vi "FTW-Test-Socket-Stress-InboxConnector.vi"() -> (0 "Test Result":errorcluster)   [LabVIEW 2014]
uses:
  src/socket/support/FTW-Socket-Core-TransportScheme.ctl
  src/error/FTW-ERR-ExceptionType.ctl
  src/error/FTW-ERR-ThrowError.vi
  lib/FTW-KernelFilepath.vi
  src/error/FTW-ERR-CallChain.vi
  src/string/FTW-STR-ReplaceWhitespace.vi
  src/json/core/FTW-JSON-Core-EncodingFlags.vi
  src/reflection/FTW-Reflection-Type.vi
  codegen/xnode/json/fetch/FTW-JSON-Core-GetFlattenedValue.vi
  src/socket/support/FTW-Socket-Core-LibraryError.vi
  src/actor/request/FTW-Request-InterpretResponse.vi
  codegen/xnode/FTW-Actor-Ask.xnode
  src/socket/connector/core/FTW-Connector-Core-Type.ctl
  codegen/xnode/FTW-JSON-Fetch.xnode
panel:
  in  "Mode":enum32{"Automated Testing", "Manual Control"}(tab)
  out "Progress":dbl(slide) scale=0.0..1.0
  in  "Test to Perform":T1(radio)=enum."Parallel: 10x100x10k"
  in  "stop":bool
  out "Results":T3(array[cluster]) {"?" format="%_3p bytes/sec (one-way receive)"; "?" format="%_3f replies/sec"; "?" format="Benchmark Time: %_3psec"}
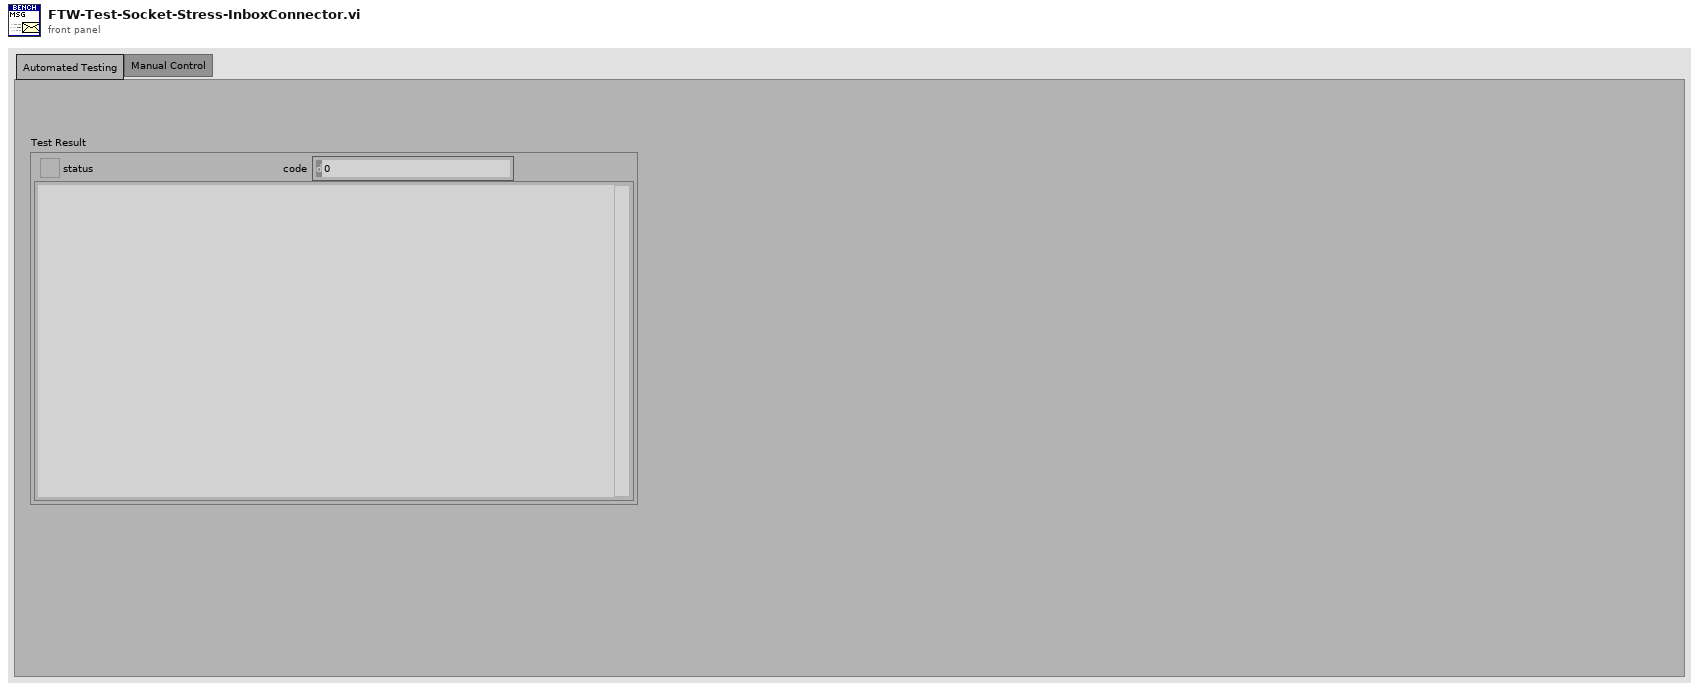
[diagram p1: front panel]
types:
  T1 = enum32{"Serial: 1x1x0", "Serial: 1x1000x0", "Serial: 1x1000x10k", "Serial: 10x100x10k", "Parallel: 10x100x10k", "Parallel: 10x10x1M", "Parallel: 100x1x10k", "Parallel: 100x100x0", "Parallel: 1000x10x1k", "Parallel: 1000x100x10k", "Parallel: 10x100x1M", "Parallel: 1000x1x1M", "Parallel: 10x10000x0"}
  T2 = typedef "FTW-Socket-Core-TransportScheme.ctl" = enum16{"TCP (tcp://)", "Inter-Process (ipc://)", "In-Process (inproc://)", "WebSocket (ws://)"}
  T3 = cluster{"Server Address":T2, "error":errorcluster, "Client Results":cluster{"Instance":string, "All replies were as expected?":bool}[], dbl, dbl, dbl, "Pass?":bool}[]
  T4 = enum32{"Serial: 1x1x0", "Serial: 1x1000x0", "Serial: 1x1000x10k", "Serial: 10x100x10k", "Parallel: 10x100x10k", "Parallel: 10x10x1M", "Parallel: 100x1x10k", "Parallel: 100x100x0", "Parallel: 1000x10x1k", "Parallel: 1000x100x10k", "Parallel: 10x100x1M", "Parallel: 1000x1x1M", "Parallel: 10x10000x0"}[]
  T5 = cluster{"Inbox Address":T2, "error out":errorcluster, cluster{string, bool}[], "Elapsed Time":dbl, dbl, dbl, bool}[]
  T6 = typedef "FTW-ERR-ExceptionType.ctl" = enum16{"OK", "Info", "Warning", "Error"}
  T7 = cluster{i32, i32, i32, i32, "Replies from Server":i32, "bytes from Server":i32, bool, bool}
  T8 = cluster{"Message Transport Scheme":T2, "error out":errorcluster, cluster{string, bool}[], "Elapsed Time":dbl, dbl, dbl, bool}
  T9 = cluster{"Message Transport Scheme":T2, "error out":errorcluster, cluster{string, bool}[], "Elapsed Time":dbl, dbl, dbl, bool}[]
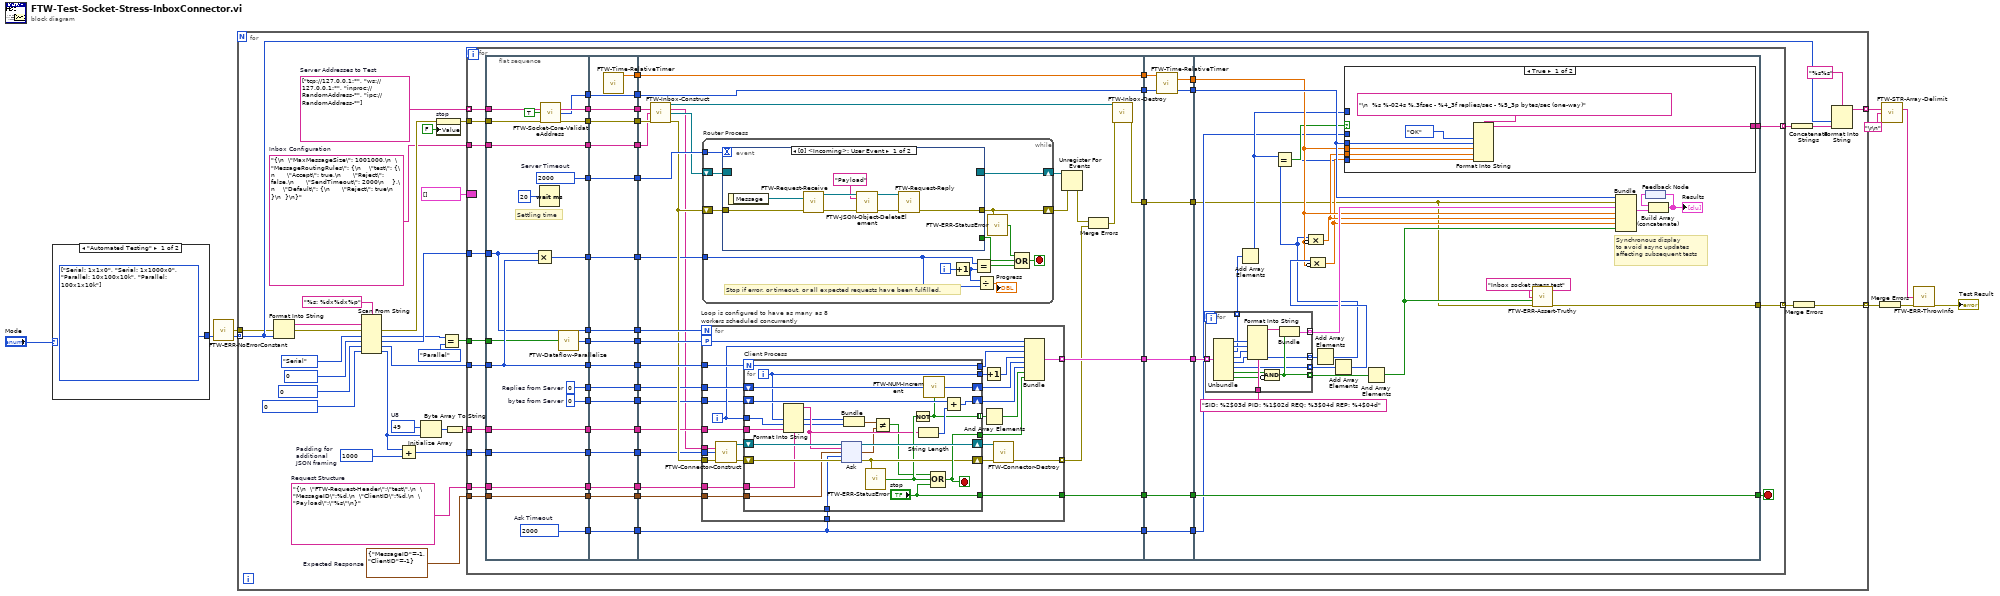
[diagram p0: block diagram]
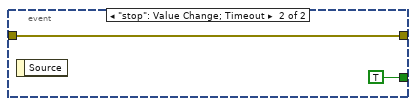
[diagram p2: hidden frame]
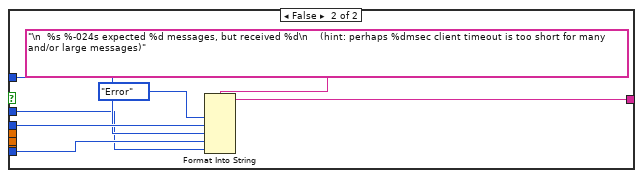
[diagram p3: hidden frame]
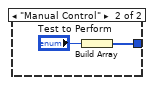
[diagram p4: hidden frame]
diagram:
  n1 = case shown="\"Automated Testing\"" "Mode" {
    tunnel: [w10 w11] -> w8
    frame "Automated Testing" {
      w10 = T4 [enum."Serial: 1x1x0", enum."Serial: 1x1000x0", enum."Parallel: 10x100x10k", enum."Parallel: 100x1x10k"] items=["Serial: 1x1x0", "Serial: 1x1000x0", "Serial: 1x1000x10k", "Serial: 10x100x10k", "Parallel: 10x100x10k", "Parallel: 10x10x1M", "Parallel: 100x1x10k", "Parallel: 100x100x0", "Parallel: 1000x10x1k", "Parallel: 1000x100x10k", "Parallel: 10x100x1M", "Parallel: 1000x1x1M", "Parallel: 10x10000x0"]
    }
    frame "Manual Control" {
      n2 = Build Array("Test to Perform") -> (w11:T4)
    }
  }
  n3 = call "FTW-ERR-NoErrorConstant.vi"() -> ("no error"=w5:errorcluster)
  n4 = for {
    tunnel: w8 -> [w24] mode=indexing
    tunnel: [w39] -> w7 mode=indexing
    tunnel: [w36] -> w3 mode=indexing
    tunnel: w5 -> [w16]
    w13 = "{\n  \"MaxMessageSize\": 1001000,\n  \"MessageRoutingRules\": {\n    \"test\": {\n      \"Accept\": true,\n      \"Reject\": false,\n      \"SendTimeout\": 2000\n    },\n    \"Default\": {\n      \"Reject\": true\n    }\n  }\n}"  # Inbox Configuration
    w14 = cluster{"MessageID":i32, "ClientID":i32} {"MessageID"=-1, "ClientID"=-1}  # Expected Response
    w15 = "{\n  \"FTW-Request-Header\":\"test\",\n  \"MessageID\":%d,\n  \"ClientID\":%d,\n  \"Payload\":\"%s\"\n}"  # Request Structure
    w20 = 1000  # Padding for additional JSON framing
    w23 = string[] ["tcp://127.0.0.1:*", "ws://127.0.0.1:*", "inproc://RandomAddress-*", "ipc://RandomAddress-*"]  # Server Addresses to Test
    w44 = u8 49  # U8
    n5 = Format Into String(error in=w16, w24) -> (resulting string=w34:string, error out=w33:errorcluster)  [unwired: 2 in]
    n6 = Scan From String(format string="%s: %dx%dx%p", input string=w34, error in=w33, default 1=enum32{"Parallel", "Serial"}."Serial", default 2=0, default 3=0, default 4=0) -> (error out=w30:errorcluster, output 1=w19:enum32{"Parallel", "Serial"}, output 2=w26:i32, output 3=w25:i32, output 4=w22:i32)  [unwired: 1 in, 2 out]
    n7 = Add(x=w22, y=w20) -> (x+y=w21:i32)
    n8 = Initialize Array(w44, w22) -> (w43:u8[])
    n9 = property on="stop" class="Bool (strict)"(error in=w30, "Value"=FALSE ("stop")) -> (error out=w45:errorcluster)  [unwired: 1 in, 1 out]
    n10 = Equal?(x=w19, y=enum32{"Parallel", "Serial"}."Parallel" ("x")) -> (x = y?=w17:bool)
    n11 = Byte Array To String(unsigned byte array=w43) -> (string=w42:string)
    n12 = for {
      tunnel: w23 -> [w97] mode=indexing
      tunnel: w26 -> [w94]
      tunnel: w25 -> [w90]
      tunnel: w45 -> [w89]
      tunnel: w42 -> [w79]
      border: T5 [] -> [_]
      tunnel: [w66] -> w40 mode=indexing
      tunnel: [w65] -> w38 mode=indexing
      tunnel: w21 -> [w57]
      tunnel: w17 -> [w56]
      tunnel: w15 -> [w53]
      tunnel: w14 -> [w52]
      tunnel: w13 -> [w47]
      stop <- w69 stop-if-true
      n13 = flat-sequence {
        tunnel: [w116] -> w104
        tunnel: [w114] -> w98
        tunnel: [w118] -> w95
        tunnel: [w124] -> w91
        tunnel: w89 -> [w117]
        tunnel: w90 -> [w124]
        tunnel: w94 -> [w118]
        tunnel: w97 -> [w115]
        tunnel: [w120] -> w87
        tunnel: [w109] -> w84
        tunnel: [w123] -> w82
        tunnel: [w122] -> w80
        tunnel: w79 -> [w122]
        tunnel: [w121] -> w77
        tunnel: [w119] -> w71
        tunnel: [w113] -> w63
        tunnel: [w111] -> w60
        tunnel: [w110] -> w58
        tunnel: w57 -> [w110]
        tunnel: w56 -> [w108]
        tunnel: [w107] -> w54
        tunnel: w53 -> [w107]
        tunnel: w52 -> [w106]
        tunnel: [w106] -> w51
        tunnel: [w105] -> w48
        tunnel: w47 -> [w105]
        tunnel: [w142] -> w103
        tunnel: [w141] -> w102
        tunnel: w104 -> [w142]
        tunnel: [w140] -> w99
        tunnel: w98 -> [w140]
        tunnel: [w139] -> w96
        tunnel: w95 -> [w139]
        tunnel: [w138] -> w92
        tunnel: w91 -> [w138]
        tunnel: [w137] -> w88
        tunnel: w87 -> [w137]
        tunnel: [w130] -> w86
        tunnel: [w136] -> w85
        tunnel: w84 -> [w136]
        tunnel: [w135] -> w83
        tunnel: w82 -> [w135]
        tunnel: [w134] -> w81
        tunnel: w80 -> [w134]
        tunnel: [w133] -> w78
        tunnel: w77 -> [w133]
        tunnel: w71 -> [w132]
        tunnel: [w132] -> w70
        tunnel: [w131] -> w64
        tunnel: w63 -> [w131]
        tunnel: w60 -> [w130]
        tunnel: [w129] -> w59
        tunnel: w58 -> [w129]
        tunnel: [w128] -> w55
        tunnel: w54 -> [w128]
        tunnel: w51 -> [w127]
        tunnel: [w127] -> w50
        tunnel: [w126] -> w49
        tunnel: w48 -> [w126]
        tunnel: [w157] -> w101
        tunnel: [w171] -> w100
        tunnel: [w170] -> w93
        tunnel: w83 -> [w155]
        tunnel: w85 -> [w164]
        tunnel: w103 -> [w163]
        tunnel: w102 -> [w171]
        tunnel: w99 -> [w162]
        tunnel: w96 -> [w166]
        tunnel: w92 -> [w167]
        tunnel: w88 -> [w165]
        tunnel: w86 -> [w147]
        tunnel: w81 -> [w156]
        tunnel: w78 -> [w153]
        tunnel: [w149] -> w72
        tunnel: w70 -> [w151]
        tunnel: [w150] -> w67
        tunnel: w64 -> [w149]
        tunnel: [w147] -> w61
        tunnel: w59 -> [w146]
        tunnel: w55 -> [w145]
        tunnel: w50 -> [w144]
        tunnel: w49 -> [w143]
        tunnel: w101 -> [w420]
        tunnel: w100 -> [w419]
        tunnel: w93 -> [w417]
        tunnel: [w420] -> w76
        tunnel: [w418] -> w75
        tunnel: [w417] -> w74
        tunnel: [w416] -> w73
        tunnel: w72 -> [w416]
        tunnel: [w415] -> w68
        tunnel: w67 -> [w415]
        tunnel: [w414] -> w62
        tunnel: w61 -> [w414]
        tunnel: w76 -> [w423]
        tunnel: w75 -> [w432]
        tunnel: w74 -> [w445]
        tunnel: w73 -> [w434]
        tunnel: [w435] -> w69
        tunnel: w68 -> [w435]
        tunnel: [w433] -> w66
        tunnel: [w422] -> w65
        tunnel: w62 -> [w425]
        frame #0 {
          w111 = 2000  # Ask Timeout
          w119 = 0  # bytes from Server
          w120 = 2000  # Server Timeout
          w121 = 0  # Replies from Server
          # "Settling time"
          n14 = Multiply(x=w118, y=w124) -> (x*y=w123:i32)
          n15 = Wait (ms)(milliseconds to wait=u32 20) -> ()  [unwired: 1 out]
          n16 = call "FTW-Socket-Core-ValidateAddress.vi"("Address"=w115, "Allow wildcard replacement?"=TRUE, "error in"=w117) -> ("Sanitized Address"=w114:string, "Message Transport Scheme"=w113:T2, "error out"=w116:errorcluster)  [unwired: 10 in]
          n17 = call "FTW-Dataflow-Parallelize.vi"("Parallelize?"=w108) -> ("Parallel Instances"=w109:i32)
        }
        frame #1 {
          n18 = call "FTW-Time-RelativeTimer.vi"() -> ("Current Timer Value"=w141:dbl)  [unwired: 13 in, 2 out]
        }
        frame #2 {
          n19 = call "FTW-Inbox-Construct.vi"("Primary Inbox Address"=w162, "Inbox Configuration"=w143, "error in"=w163) -> ("FTW Router"=w161:refnum<data-value>, "Resolved Primary Inbox Address"=w148:string, "Incoming Request"=w154:refnum<event-registration>, "error out"=w160:errorcluster)  [unwired: 9 in]
          n20 = for "Loop is configured to have as many as 8 workers scheduled concurrently" {
            N: w166 -> [_]
            tunnel: w160 -> [w177]
            tunnel: w167 -> [w198]
            tunnel: w147 -> [w197]
            workers-P: w164 -> [w194]
            tunnel: [w196] -> w170 mode=indexing
            tunnel: w148 -> [w178]
            tunnel: [w190] -> w152 mode=indexing
            tunnel: w156 -> [w188]
            tunnel: w153 -> [w187]
            tunnel: w151 -> [w182]
            tunnel: [w180] -> w150
            tunnel: w146 -> [w173]
            tunnel: w145 -> [w174]
            tunnel: w144 -> [w172]
            i -> [w185]
            n21 = call "FTW-Connector-Construct.vi"("Remote Inbox Address"=w178, "Receive Message Size Limit"=w173, "error in"=w177) -> ("FTW Actor Connector"=w175:refnum<data-value>, "error out"=w176:errorcluster)  [unwired: 11 in]
            n22 = for "Client Process" {
              N: w198 -> [w210]
              shift-right: [w221] -> w192
              shift-left: w175 -> [w222]
              tunnel: w197 -> [w217]
              tunnel: [w220] -> w195
              tunnel: [w209] -> w189 mode=indexing
              shift-right: [w218] -> w191
              shift-left: w176 -> [w219]
              tunnel: w185 -> [w202]
              tunnel: w188 -> [w207]
              shift-right: [w216] -> w186
              shift-left: w187 -> [w215]
              tunnel: [w203] -> w184
              shift-right: [w213] -> w181
              shift-left: w182 -> [w212]
              tunnel: ["stop"] -> w180
              tunnel: [w210] -> w179
              tunnel: w174 -> [w206]
              tunnel: w172 -> [w204]
              i -> [w203]
              stop <- w220 stop-if-true
              n23 = Format Into String(format string=w206, w203, w202, w207) -> (resulting string=w205:string)  [unwired: 2 in, 1 out]
              n24 = xnode "Ask"("FTW Actor Connector"=w222, "Request"=w205, "Response Type and Defaults"=w204, "Timeout"=w217, "error in"=w219) -> ("FTW Actor Connector out"=w221:refnum<data-value>, "Response"=w200:cluster{"MessageID":i32, "ClientID":i32}, "error out"=w218:errorcluster)  [unwired: 1 out]
              n25 = Bundle(w203, w202) -> (w201:cluster{i32, i32})  [unwired: 1 in]
              n26 = call "FTW-ERR-StatusError.vi"("error to check"=w218) -> ("Error?"=w208:bool)
              n27 = Not Equal?(x=w201, y=w200) -> (x != y?=w199:bool)
              n28 = Not(x=w208) -> (.not. x?=w209:bool)
              n29 = String Length(string=w205) -> (length=w214:i32)
              n30 = call "FTW-NUM-Increment.vi"("Initial Value"=w215, "Increment?"=w209) -> ("Final Value"=w216:i32)
              n31 = Compound Arithmetic op=OR(w199, w208, "stop") -> (w220:bool)
              n32 = Add(x=w212, y=w214) -> (x+y=w213:i32)
            }
            n33 = Increment(x=w184) -> (x+1=w183:i32)
            n34 = And Array Elements(Boolean array=w189) -> (logical AND=w193:bool)
            n35 = call "FTW-Connector-Destroy.vi"("FTW Connector"=w192, "error in"=w191) -> ("error out"=w190:errorcluster)  [unwired: 13 in]
            n36 = Bundle(w194, w185, w179, w183, "Replies from Server"=w186, "bytes from Server"=w181, w193, w195) -> (w196:T7)  [unwired: 1 in]
          }
          n37 = while "Router Process" {
            shift-right: [w402] -> w168
            shift-left: w154 -> [w403]
            shift-right: [w400] -> w169
            shift-left: w160 -> [w401]
            tunnel: w155 -> [w393]
            tunnel: w165 -> [w395]
            i -> [w394]
            stop <- w396 stop-if-true
            # "Stop if error, or timeout, or all expected requests have been fulfilled."
            n38 = event shown="[0] <Incoming>: User Event" {
              selector: w403 -> [_ _]
              dyn-events: [_ _] -> w402
              timeout: w395 -> [_ _]
              tunnel: [_ TRUE] -> w398
              tunnel: w401 -> [w409 w412]
              tunnel: [w411 w412] -> w400
              event User Event {
                n39 = event-data() -> ("Message"=w410:refnum<queue>)  [unwired: 1 in]
                n40 = call "FTW-Request-Receive.vi"("MessagePipe"=w410, "error in"=w409) -> ("Request"=w408:refnum<data-value>, "error out"=w406:errorcluster)  [unwired: 11 in, 1 out]
                n41 = call "FTW-JSON-Object-DeleteElement.vi"("JSON Object"=w408, "Key"="Payload", "error in"=w406) -> ("JSON Object out"=w407:refnum<data-value>, "error out"=w405:errorcluster)  [unwired: 10 in, 1 out]
                n42 = call "FTW-Request-Reply.vi"("Request"=w407, "error in"=w405) -> ("error out"=w411:errorcluster)  [unwired: 13 in]
              }
              event "stop": Value Change; Timeout {
                n43 = event-data() -> ()  [unwired: 1 in, 1 out]
              }
            }
            n44 = Increment(x=w394) -> (x+1=w392:i32)
            n45 = Equal?(x=w393, y=w392) -> (x = y?=w397:bool)
            n46 = Divide(x=w392, y=w393) -> (x/y=→"Progress":dbl)
            n47 = call "FTW-ERR-StatusError.vi"("error to check"=w400) -> ("Error?"=w399:bool)
            n48 = Compound Arithmetic op=OR(w399, w398, w397) -> (w396:bool)
          }
          n49 = Unregister For Events(event registration refnum=w168, error in=w169) -> (error out=w159:errorcluster)
          n50 = Merge Errors(w159, w152) -> (w158:errorcluster)
          n51 = call "FTW-Inbox-Destroy.vi"("FTW Router"=w161, "error in"=w158) -> ("error out"=w157:errorcluster)  [unwired: 13 in]
        }
        frame #3 {
          n52 = call "FTW-Time-RelativeTimer.vi"("Previous Timer Value"=w419) -> ("Elapsed Time"=w418:dbl)  [unwired: 12 in, 2 out]
        }
        frame #4 {
          # "Synchronous display\nto avoid async updates\naffecting subsequent tests"
          n53 = for {
            tunnel: w445 -> [w472] mode=indexing
            tunnel: "SID: %2$03d PID: %1$02d REQ: %3$04d REP: %4$04d" -> [w471]
            tunnel: [w467] -> w442 mode=indexing
            tunnel: [w466] -> w444 mode=indexing
            tunnel: [w463] -> w440 mode=indexing
            tunnel: [w462] -> w436 mode=indexing
            tunnel: [w460] -> w429 mode=indexing
            n54 = Unbundle(w472) -> (w470:i32, w469:i32, w460:i32, w461:i32, "Replies from Server"=w462:i32, "bytes from Server"=w463:i32, w464:bool, w465:bool)
            n55 = Format Into String(format string=w471, w470, w469, w461, w462) -> (resulting string=w468:string)  [unwired: 2 in, 1 out]
            n56 = Compound Arithmetic op=AND(w464, invert w465) -> (w466:bool)
            n57 = Bundle(w468, w466) -> (w467:cluster{string, bool})  [unwired: 1 in]
          }
          n58 = Add Array Elements(numeric array=w429) -> (sum=w427:i32)
          n59 = Add Array Elements(numeric array=w436) -> (sum=w426:i32)
          n60 = Equal?(x=w427, y=w426) -> (x = y?=w428:bool)
          n61 = Compound Arithmetic op=MULTIPLY(w426, invert w432) -> (w431:dbl)
          n62 = Add Array Elements(numeric array=w440) -> (sum=w437:i32)
          n63 = Compound Arithmetic op=MULTIPLY(w437, invert w432) -> (w430:dbl)
          n64 = case shown="True" w428 {
            tunnel: w434 -> [w452 w459]
            tunnel: [w450 w457] -> w433
            tunnel: w432 -> [w449 _]
            tunnel: w431 -> [w448 _]
            tunnel: w430 -> [w447 _]
            tunnel: w427 -> [_ w456]
            tunnel: w426 -> [_ w455]
            tunnel: w425 -> [_ w454]
            frame True {
              n65 = Format Into String(format string="\n  %s %-024s %.3fsec - %4_3f replies/sec - %5_3p bytes/sec (one-way)", FTW-ERR-ExceptionType."OK" ("Exception"), w452, w449, w448, w447) -> (resulting string=w450:string)  [unwired: 2 in, 1 out]
            }
            frame False {
              n66 = Format Into String(format string="\n  %s %-024s expected %d messages, but received %d\n    (hint: perhaps %dmsec client timeout is too short for many and/or large messages)", FTW-ERR-ExceptionType."Error" ("Exception"), w459, w456, w455, w454) -> (resulting string=w457:string)  [unwired: 2 in, 1 out]
            }
          }
          n67 = And Array Elements(Boolean array=w444) -> (logical AND=w424:bool)
          n68 = call "FTW-ERR-Assert-Truthy.vi"("Assertion"="Inbox socket stress test", "Assertion holds true?"=w424, "error in"=w423) -> ("error out"=w422:errorcluster)  [unwired: 12 in]
          n69 = Bundle("Message Transport Scheme"=w434, "error out"=w423, w442, "Elapsed Time"=w432, w431, w430, w424) -> (w439:T8)  [unwired: 1 in]
          n70 = feedback #1() -> (w443:T5)
          n71 = Build Array (concatenate)(w443, w439) -> (w438:T9)
          "Results" <- w438
          n72 = feedback-in #1(w438) -> ()
        }
      }
    }
    n73 = Concatenate Strings(w40) -> (w37:string)
    n74 = Merge Errors(w38) -> (w39:errorcluster)
    n75 = Format Into String(format string="%s%s", w24, w37) -> (resulting string=w36:string)  [unwired: 2 in, 1 out]
  }
  n76 = Merge Errors(w7) -> (w4:errorcluster)
  n77 = call "FTW-STR-Array-Delimit.vi"("Array of Strings"=w3, "Delimiter"="\r\n") -> ("Delimited String"=w2:string)  [unwired: 13 in]
  n78 = call "FTW-ERR-ThrowInfo.vi"("Informational Message"=w2, "error in"=w4) -> ("error out"=→"Test Result":errorcluster)  [unwired: 13 in]
